vi "startPopup.vi"() -> (1 "Bearbeiter":string, 2 "OBNr":string, 3 "Baugruppe":string)   [LabVIEW 2013]
panel:
  in  "OK Button":bool
  in  "Orderbase Nr.":string
  in  "Bearbeiter":string
  in  "Name Baugruppe":string
  # "EMV - Prüfung"
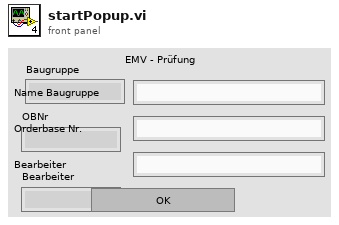
[diagram p1: front panel]
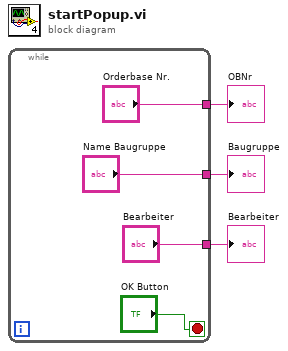
[diagram p0: block diagram]
diagram:
  n1 = while {
    tunnel: ["Name Baugruppe"] -> w3
    tunnel: ["Orderbase Nr."] -> w2
    tunnel: ["Bearbeiter"] -> w1
    stop <- "OK Button" stop-if-true
  }
  "Baugruppe" <- w3
  "OBNr" <- w2
  "Bearbeiter" <- w1
